vi "WT-Voltage-Controller-Current-No-Log.vi"() -> ()   [LabVIEW 2017]
uses:
  <vilib>/Platform/TimedLoop/XDataNode/timing_clust.ctl
  <vilib>/Platform/TimedLoop/XDataNode/nitl_modes.ctl
  <vilib>/Platform/TimedLoop/XDataNode/wakeup.ctl
  <vilib>/DAQmx/read.llb/DAQmx Read (Analog 1D DBL NChan 1Samp).vi
  <vilib>/Analysis/baseanly.llb/Mean (DBL).vi
  <vilib>/DAQmx/miscellaneous.llb/DAQmx Fill In Error Info.vi
  <vilib>/platform/TimedLoop/XDataNode/XDataNode.xnode
  <vilib>/Platform/TimedLoop/XDataNode/XDNodeRunTimeDep.lvlib
  <vilib>/Analysis/NI_AALBase.lvlib
panel:
  out "Fan 2 (A)":dbl format="%0.2f"
  out "Fan 1 (A)":dbl format="%0.2f"
  out "Boolean":bool
  in  "POWER":bool
  in  "Sync":bool
  out "error out":errorcluster
  in  "Fan 2 Voltage":dbl
  in  "Fan 1 Voltage":dbl
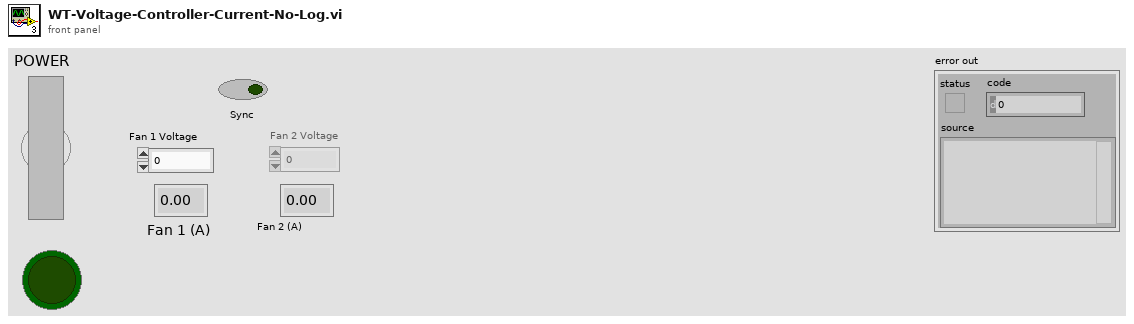
[diagram p1: front panel]
types:
  T1 = typedef "XDNodeRunTimeDep.lvlib/timing_clust.ctl" = cluster{"Expected End [f-1]":u64, "Actual End [f-1]":u64, "Finished Late? [f-1]":bool, "Expected End [i-1]":u64, "Actual End [i-1]":u64, "Finished Late? [i-1]":bool, "Expected Start [i]":u64, "Actual Start [i]":u64, "Expected Start [f]":u64, "Actual Start [f]":u64, "Source Name":string, "Structure Name":string, "Period":i64, "Deadline":i64, "Offset":i64, "Start":i64, "Priority":i32, "Timeout":i32, "Mode":T2, "Wakeup Reason":T3, "Error":errorcluster, "Source Type":string, "Secondary Source Type":string, "Global End Time":u64, "Global Start Time":u64, "Frame Duration":u64, "Iteration Duration":u64, "Assigned CPU":i32, "I/O Scan Engine Mode":u32}
  T2 = typedef "XDNodeRunTimeDep.lvlib/nitl_modes.ctl" = enum32{"No Change", "Process missed periods, maintain original phase", "Discard missed periods, maintain original phase", "Process missed periods, ignore original phase", "Discard missed periods, ignore original phase"}
  T3 = typedef "XDNodeRunTimeDep.lvlib/wakeup.ctl" = enum32{"Normal", "Aborted", "Asynchronous wakeup", "Timing source error", "Timed loop error", "Timeout"}
  T4 = enum8{"Enabled", "Disabled", "Disabled and Grayed Out"}
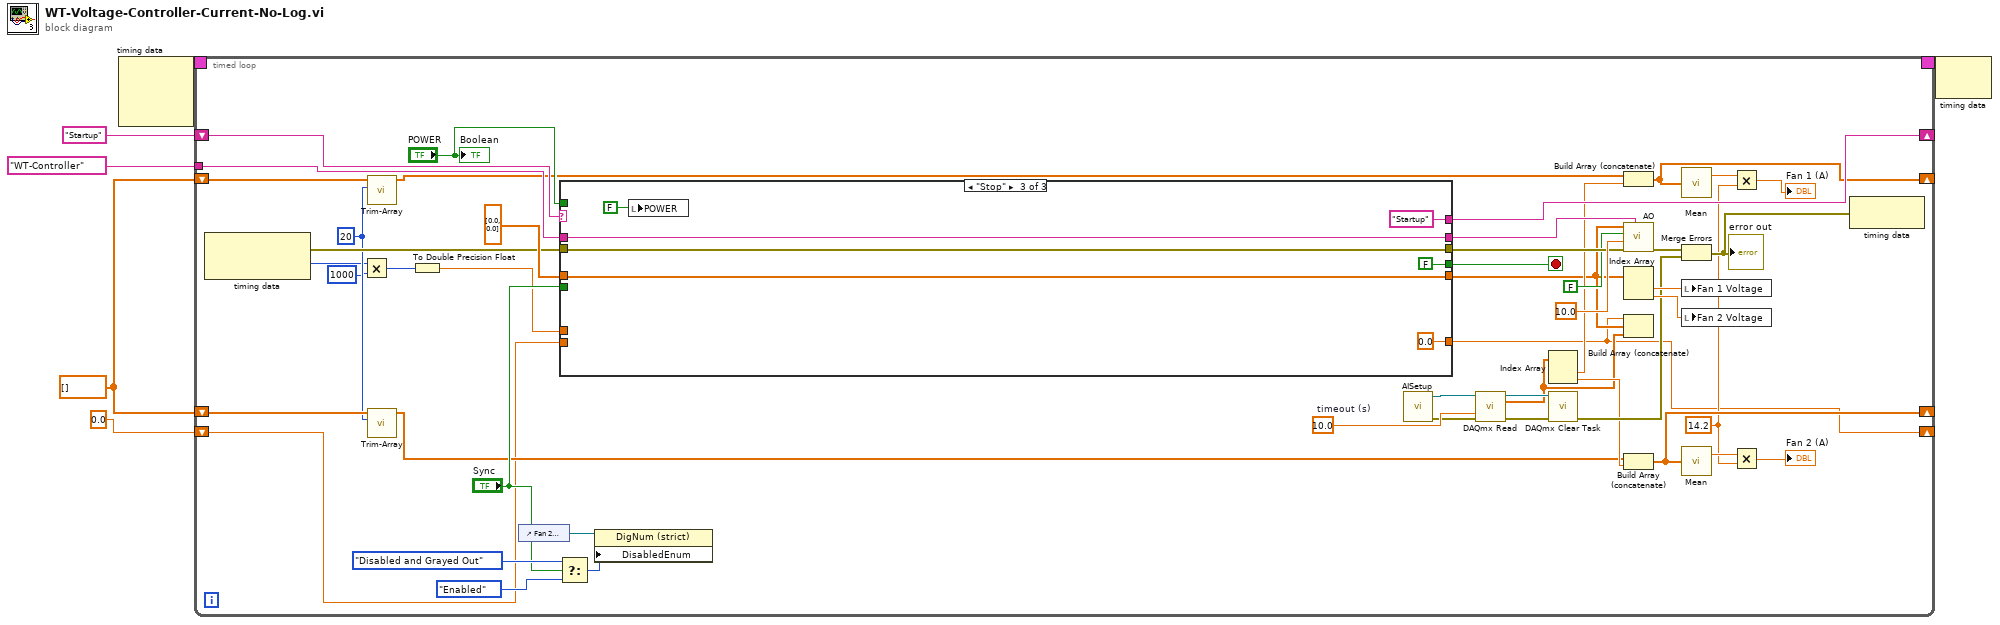
[diagram p0: block diagram]
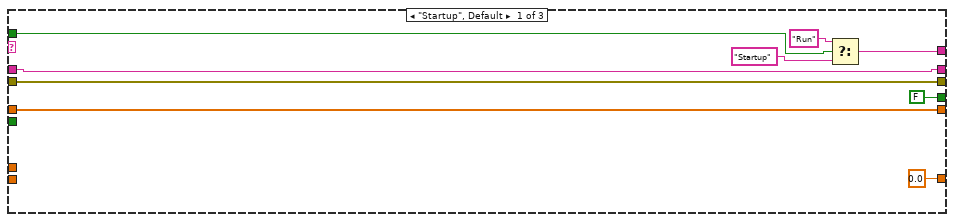
[diagram p2: hidden frame]
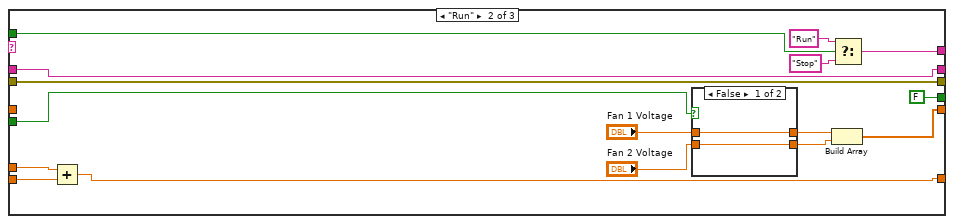
[diagram p3: hidden frame]
diagram:
  w2 = dbl[] []
  n1 = node-c288() -> (w4:T1)  [unwired: 3 in]
  n2 = timed-loop {
    shift-right: [w53] -> _
    shift-left: "Startup" -> [w54]
    tunnel: tag "WT-Controller" ("device name") -> [w51]
    timing: w4 -> [_]
    timing-out: [_] -> w3
    shift-right: [w25] -> _
    shift-left: w2 -> [w23]
    shift-right: [w24] -> _
    shift-left: w2 -> [w22]
    shift-right: [w7] -> _
    shift-left: 0.0 -> [w9]
    stop <- w52 stop-if-true
    w16 = 14.2 ("y")
    w20 = 20 ("length")
    w36 = 10.0  # timeout (s)
    n3 = node-c288() -> (w41:errorcluster, w12:i64)  [unwired: 1 in]
    n4 = Multiply(x=w12, y=i64 1000) -> (x*y=w10:i64)
    n5 = call "Trim-Array.vi"("length"=w20, "Array in"=w23) -> ("Array out"=w27:dbl[])  [unwired: 9 in]
    n6 = call "Trim-Array.vi"("length"=w20, "Array in"=w22) -> ("Array out"=w21:dbl[])  [unwired: 9 in]
    n7 = To Double Precision Float(number=w10) -> (double precision float=w8:dbl)
    n8 = control-ref of="Fan 2 Voltage"() -> (w47:refnum<vi>)
    n9 = case shown="\"Stop\"" w54 {
      tunnel: [w63 w85 "Startup" ("f")] -> w53
      tunnel: [w68 w78 w93] -> w14
      tunnel: [FALSE ("Stop") FALSE ("Stop") FALSE ("Stop")] -> w52
      tunnel: w51 -> [w67 w77 w94]
      tunnel: [w69 w76 w92] -> w43
      tunnel: w41 -> [w69 w76 w92]
      tunnel: "Sync" -> [_ w80 _]
      tunnel: dbl[] [0.0, 0.0] ("appended array") -> [w68 _ w93]
      tunnel: [w67 w77 w94] -> w42
      tunnel: "POWER" -> [w65 w75 _]
      tunnel: w9 -> [_ w72 _]
      tunnel: [0.0 w70 0.0] -> w7
      tunnel: w8 -> [_ w71 _]
      frame "Startup", Default {
        n10 = Select(t="Run" ("f"), s=w65, f="Startup") -> (s? t:f=w63:string)
      }
      frame "Run" {
        n11 = Add(x=w71, y=w72) -> (x+y=w70:dbl)
        n12 = case shown="False" w80 {
          tunnel: [w86 w88] -> w83
          tunnel: [w87 w88] -> w82
          tunnel: "Fan 1 Voltage" -> [w87 w88]
          tunnel: "Fan 2 Voltage" -> [w86 _]
          frame False {
          }
          frame True {
          }
        }
        n13 = Build Array(w82, w83) -> (w78:dbl[])
        n14 = Select(t="Run" ("f"), s=w75, f="Stop") -> (s? t:f=w85:string)
      }
      frame "Stop" {
        n15 = local write "POWER"(FALSE ("POWER")) -> ()
      }
    }
    n16 = Select(t=T4."Disabled and Grayed Out" ("Disabled"), s="Sync", f=T4."Enabled") -> (s? t:f=w49:T4)
    n17 = property class="DigNum (strict)"(reference=w47, "DisabledEnum"=w49) -> ()  [unwired: 1 in, 2 out]
    n18 = call "AISetup.vi"() -> ("error out"=w32:errorcluster, "task out"=w33:refnum<k21>)  [unwired: 10 in]
    n19 = call-poly <vilib>:"DAQmx Read.vi"("task/channels in"=w33, "timeout"=w36, "error in"=w32) -> ("task out"=w34:refnum<k21>, "data"=w13:dbl[], "error out"=w35:errorcluster)  [unwired: 10 in]
    n20 = Index Array(array=w13) -> (element #1=w28:dbl, element #2=w26:dbl)  [unwired: 2 in]
    n21 = call <vilib>:"DAQmx Clear Task.vi"("task in"=w34, "error in"=w35) -> ("error out"=w31:errorcluster)  [unwired: 13 in]
    n22 = Build Array (concatenate)(w27, w28) -> (w25:dbl[])
    n23 = call "AO.vi"("device name"=w42, "error in"=w43, "timeout (s)"=10.0, "stop (T)"=FALSE, "data"=w14) -> ("error out"=w30:errorcluster)  [unwired: 2 in, 1 out]
    n24 = Index Array(array=w14) -> (element #1=w40:dbl, element #2=w39:dbl)  [unwired: 2 in]
    n25 = Build Array (concatenate)(w7, w14, w13) -> ()  [unwired: 1 out]
    n26 = Build Array (concatenate)(w21, w26) -> (w24:dbl[])
    n27 = call-poly <vilib>:"Mean.vi"("X"=w25) -> ("mean"=w19:dbl)  [unwired: 1 out]
    n28 = Merge Errors(w30, w31) -> (w29:errorcluster)
    "error out" <- w29
    n29 = local write "Fan 1 Voltage"(w40) -> ()
    n30 = local write "Fan 2 Voltage"(w39) -> ()
    n31 = call-poly <vilib>:"Mean.vi"("X"=w24) -> ("mean"=w17:dbl)  [unwired: 1 out]
    n32 = Multiply(x=w19, y=w16) -> (x*y=→"Fan 1 (A)":dbl)
    n33 = Multiply(x=w17, y=w16) -> (x*y=→"Fan 2 (A)":dbl)
    n34 = node-c288(w29) -> ()  [unwired: 1 out]
    "Boolean" <- "POWER"
  }
  n35 = node-c288(w3) -> ()  [unwired: 1 out]
